vi "UsrProfiles-Set user button.vi"(8 "error in (no error)":errorcluster) -> (0 "error out":errorcluster)   [LabVIEW 2013]
uses:
  Global Variables/gl_UI Ctrl Refs.vi
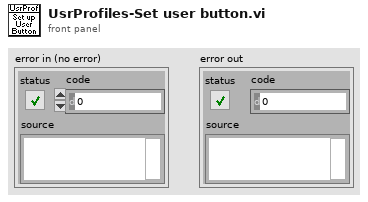
[diagram p1: front panel]
types:
  T1 = typedef "UI ctrl refs cluster.ctl" = cluster{"Top level VI path":path, "Top level VI ref":refnum<vi>, "User menu ref":refnum<k9>, "Sub Panel control":refnum<vi>, "Imaging Param Tab":refnum<vi>, "Occurrence-Start drivers":refnum<k4>, "Occurrence-Speed logging initialised":refnum<k4>, "Occurrence-XYZ stage initialised":refnum<k4>, "Exit button":refnum<vi>, "Status ind":refnum<vi>, "Return to Origin":refnum<vi>, "Speed Logging":refnum<vi>, "Time Lapse":refnum<vi>, "Live Imaging":refnum<vi>, "AOL Z Stack":refnum<vi>, "Motor Z Stack":refnum<vi>, "Funct Acq button":refnum<vi>, "Hard Shutter":refnum<vi>, "Virtual Shutter":refnum<vi>, "Laser Power":refnum<vi>, "AOL Mode":refnum<vi>, "Frame Size":refnum<vi>, "Field of View":refnum<vi>, "Dwell Time":refnum<vi>, "Zoom":refnum<vi>, "AOL Z":refnum<vi>, "Objective":refnum<vi>, "Axis":refnum<vi>, "Paths & Names":refnum<vi>, "Experiment folder path (ind.)":refnum<vi>, "Last State (Ind.)":refnum<vi>, "Laser wavelength ind (nm)":refnum<vi>, "Averages":refnum<vi>, "Angle (degrees)":refnum<vi>, "X centre":refnum<vi>, "Y centre":refnum<vi>, "Plane Mode":refnum<vi>, "# Planes":refnum<vi>, "Z Start":refnum<vi>, "Z Stop":refnum<vi>, "Z Step":refnum<vi>, "PMT 1":refnum<vi>, "PMT 2":refnum<vi>, "Stage XYZ Position":refnum<vi>, "Pockels@Z Start":refnum<vi>, "Pockels@Z Stop":refnum<vi>, "Obtain Z Start":refnum<vi>, "Obtain Z Stop":refnum<vi>, "Live stim.trig.period":refnum<vi>, "Live stim.trig.enable":refnum<vi>, "Funct. Acq. Pockels Modulation":refnum<vi>, "Enable Video Recording":refnum<vi>, "Video Record-Live Imaging":refnum<vi>, "Video Record-Funct acq":refnum<vi>, "AOL Z-stack Chirps Ready (ind)":refnum<vi>, "Center freq ind (nm)":refnum<vi>, "Logging queue (ind)":refnum<vi>, "Back aperture power (ind.)":refnum<vi>, "Power after objective (ind.)":refnum<vi>, "Switch user":refnum<vi>}
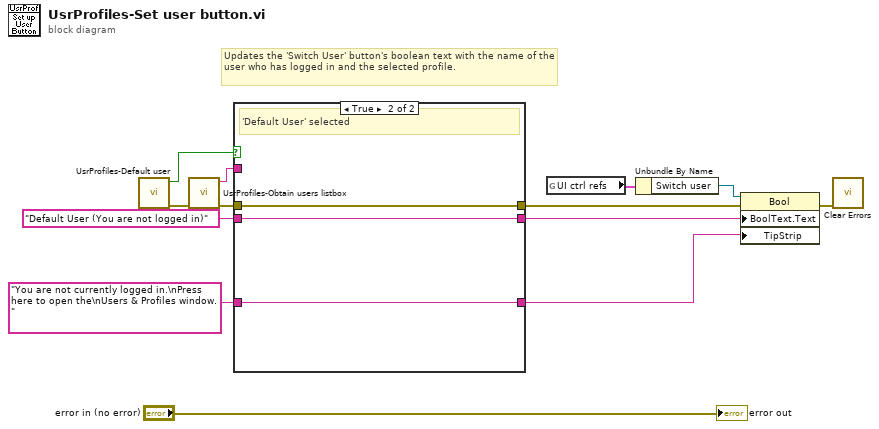
[diagram p0: block diagram]
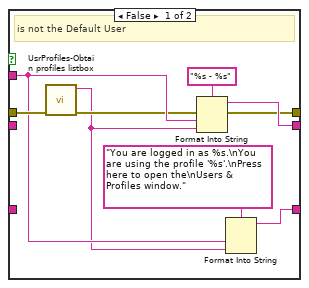
[diagram p2: hidden frame]
diagram:
  # "Updates the 'Switch User' button's boolean text with the name of the user who has logged in and the selected profile."
  n1 = call "UsrProfiles-Default user.vi"() -> ("error out"=w1:errorcluster, "Default user selected"=w2:bool)  [unwired: 9 in, 1 out]
  n2 = call "UsrProfiles-Obtain users listbox.vi"("error in (no error)"=w1) -> ("error out"=w4:errorcluster, "Selected user's name"=w3:string)  [unwired: 7 in, 2 out]
  n3 = case shown="True" w2 {
    tunnel: [w17 w24] -> w8
    tunnel: w4 -> [w22 w23]
    tunnel: [w15 w23] -> w13
    tunnel: w3 -> [w18 _]
    tunnel: [w20 w25] -> w6
    tunnel: "You are not currently logged in.\nPress here to open the\nUsers & Profiles window." ("Tip Strip") -> [_ w25]
    tunnel: "Default User (You are not logged in)" -> [_ w24]
    frame False {
      # "is not the Default User"
      n4 = call "UsrProfiles-Obtain profiles listbox.vi"("error in (no error)"=w22) -> ("error out"=w16:errorcluster, "Selected profile's name"=w14:string)  [unwired: 7 in, 2 out]
      n5 = Format Into String(format string="%s - %s", error in=w16, w18, w14) -> (resulting string=w17:string, error out=w15:errorcluster)  [unwired: 1 in]
      n6 = Format Into String(format string="You are logged in as %s.\nYou are using the profile '%s'.\nPress here to open the\nUsers & Profiles window." ("Tip Strip"), w18, w14) -> (resulting string=w20:string)  [unwired: 2 in, 1 out]
    }
    frame True {
      # "'Default User' selected"
    }
  }
  n7 = global read "gl_UI Ctrl Refs.vi" "UI ctrl refs"() -> (w12:T1)
  n8 = Unbundle By Name(w12) -> ("Switch user"=w11:refnum<vi>)
  n9 = property class="Bool"(reference=w11, error in=w13, "BoolText.Text"=w8, "TipStrip"=w6) -> (error out=w9:errorcluster)  [unwired: 1 out]
  n10 = call <vilib>:"Clear Errors.vi"("error in (no error)"=w9) -> ()  [unwired: 6 in, 1 out]
  "error out" <- "error in (no error)"
